vi "1. Empty String to Typical data types.vi"() -> ()   [LabVIEW 2017]
doc: "### Overview\nDemonstrates how the CSM API supports converting empty strings to typical data types. In most cases, an empty string is converted to the numerical value connected to the reference data type. The following is an exception:\n\n- **String data type:** An empty string converts to an empty string.\n\n### Introduction\nDemonstrates converting various empty strings to typical data types. Pay special attention to the exception regarding the String data type. The front panel displays the reference values and the converted values for comparison.\n### Steps\n\n- step1: For all common types, an empty string converts to the numerical value connected to the reference data type.\n- step2: For the String data type, an empty string converts to an empty string.\n- step3: For the Timestamp data type, an empty string converts to the current time."
uses:
  2bb2f873-33e8-4fbc-8df2-f8c3b892e92f.vi
  d59d594f-6358-4fe9-a0ea-ade5f599e91a.vi
  177f037c-d6c1-4684-97ba-f775e359171c.vi
  f8914412-5770-4d7c-8ed9-34d3b6c64140.vi
  83982d16-e29d-493a-892c-93b6b063dd3a.vi
  40fc1cc9-77e3-4a14-9bb9-de70462c7f35.vi
  81b41104-5ca5-45e9-a143-87b761583821.vi
  38ed8c4c-bfe5-4ceb-af5c-8de10cee5e52.vi
  a345cc07-d10f-4275-8a18-17707c3f89e9.vi
  cabc4c38-4671-4b03-9489-31c074b0dc0c.vi
  efc68658-e21b-4998-9bfe-a9de0054dd82.vi
  0842be61-58c2-4c06-9355-20aaf40be817.vi
  a49a9376-e1ff-4fda-bff8-7fdb6b491f6f.vi
  addons/API-String-Arugments-Support/_Support/Convert API String Arguments to Data(variant).vi
panel:
  out "timestamp":T1={"Argument String"="", "Type"=timestamp(0 s since 1904-01-01), "Retrieved TimeStamp"=timestamp(3839278850.481537 s since 1904-01-01)}
  out "2d double array":T2={"Empty API String"="", "2D DBL"=[[3.12, 4.113, 2.3, 5.0, 5.0, 2.3, 4.11, 5.0]], "Retrieved Data"=[[3.12, 4.113, 2.3, 5.0, 5.0, 2.3, 4.11, 5.0]]}
  out "cluster array":T3={"Empty API String"="", "Cluster Array"=[{"Name"="", "Child"={"Name"="ddd"}, "Bool"=FALSE}, {"Name"="ddd", "Child"={"Name"=""}, "Bool"=TRUE}], "Retrieved Data"=[{"Name"="", "Child"={"Name"="ddd"}, "Bool"=FALSE}, {"Name"="ddd", "Child"={"Name"=""}, "Bool"=TRUE}]}
  out "cluster":T4={"Empty API String"="", "Cluster"={"Name"="abc", "Child"={"Name"="ddd"}, "Bool"=FALSE}, "Retrieved Data"={"Name"="abc", "Child"={"Name"="ddd"}, "Bool"=FALSE}}
  out "1d dbl":T5={"Empty API String"="", "1D DBL"=[3.12, 4.11, 5.0], "Retrieved Data"=[3.12, 4.11, 5.0]}
  out "enum3":T6={"Empty API String"="", "Enum"=enum."2 - bbbb", "Retrieved Data"=enum."1 - aaaa"}
  out "enum2":T6
  out "enum1":T7={"Empty API String"="", "Enum"=enum."ccccc", "Retrieved Data"=enum."aaaa"}
  out "dbl":T8={"Empty API String"="", "DBL"=3.1415926, "Retrieved Data"=3.1415926}
  out "i32":T9={"Empty API String"="", "I32"=66, "Retrieved Data"=66}
  out "boolean":T10={"Empty API String"="", "Boolean"=TRUE, "Retrieved Data"=TRUE}
  out "string":T11={"Empty API String"="", "String"="abcd", "Retrieved Data"=""}
  out "path":T12={"Empty API String"="", "Path"=path "C:/ni-rt/data/a/2023.07.25", "Retrieved Data"=path "C:/ni-rt/data/a/2023.07.25"}
  # "#CSM-Example Overview\nDemonstrates how the CSM API supports converting empty strings to typical data types. In most cases, an empty string is converted to the numerical value connected to the reference data type. The following is an exception:\n\n- **String data type:** An empty string converts to an empty string."
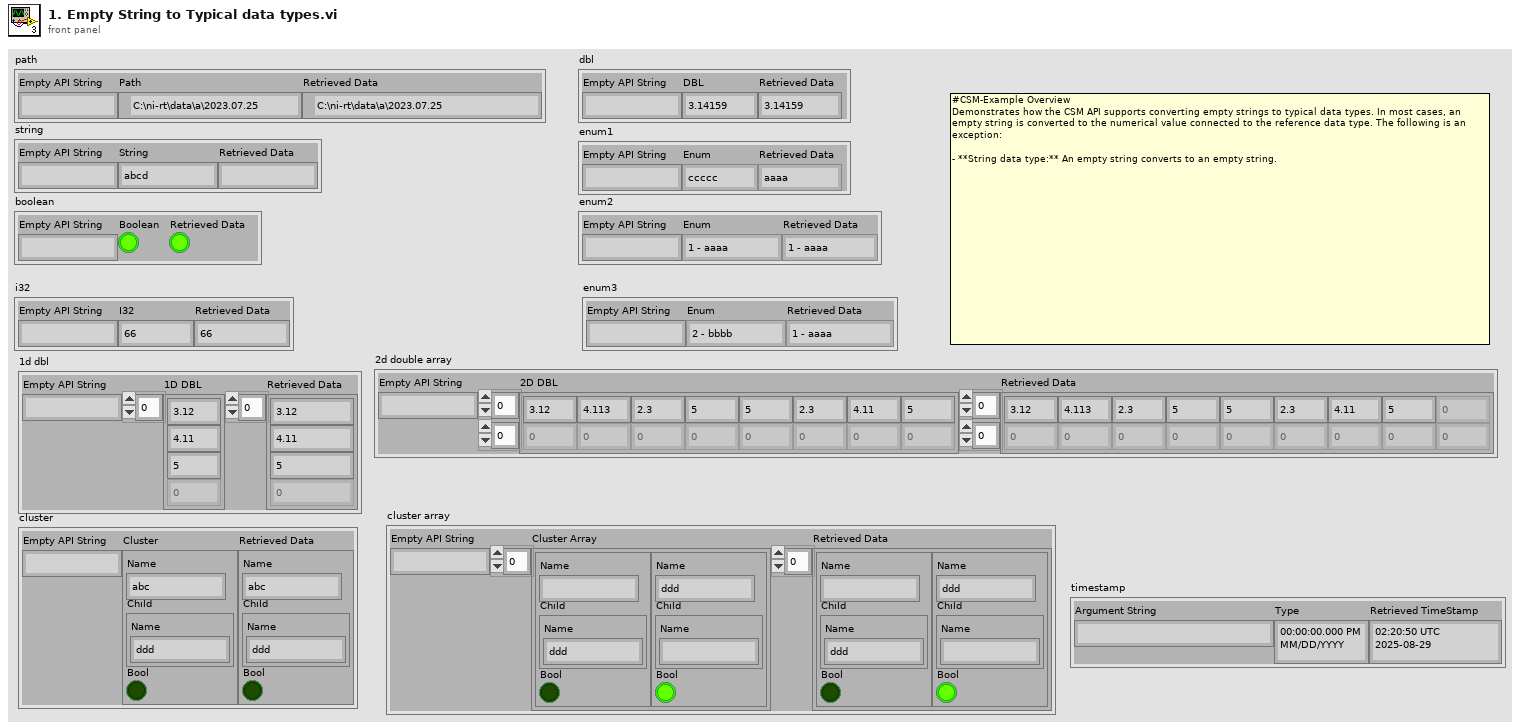
[diagram p1: front panel]
types:
  T1 = cluster{"Argument String":string, "Type":timestamp, "Retrieved TimeStamp":timestamp}
  T2 = cluster{"Empty API String":string, "2D DBL":dbl[][], "Retrieved Data":dbl[][]}
  T3 = cluster{"Empty API String":string, "Cluster Array":cluster{"Name":string, "Child":cluster{"Name":string}, "Bool":bool}[], "Retrieved Data":cluster{"Name":string, "Child":cluster{"Name":string}, "Bool":bool}[]}
  T4 = cluster{"Empty API String":string, "Cluster":cluster{"Name":string, "Child":cluster{"Name":string}, "Bool":bool}, "Retrieved Data":cluster{"Name":string, "Child":cluster{"Name":string}, "Bool":bool}}
  T5 = cluster{"Empty API String":string, "1D DBL":dbl[], "Retrieved Data":dbl[]}
  T6 = cluster{"Empty API String":string, "Enum":enum16{"1 - aaaa", "2 - bbbb", "555 - ccccc"}, "Retrieved Data":enum16{"1 - aaaa", "2 - bbbb", "555 - ccccc"}}
  T7 = cluster{"Empty API String":string, "Enum":enum16{"aaaa", "bbbb", "ccccc"}, "Retrieved Data":enum16{"aaaa", "bbbb", "ccccc"}}
  T8 = cluster{"Empty API String":string, "DBL":dbl, "Retrieved Data":dbl}
  T9 = cluster{"Empty API String":string, "I32":i32, "Retrieved Data":i32}
  T10 = cluster{"Empty API String":string, "Boolean":bool, "Retrieved Data":bool}
  T11 = cluster{"Empty API String":string, "String":string, "Retrieved Data":string}
  T12 = cluster{"Empty API String":string, "Path":path, "Retrieved Data":path}
  T13 = cluster{"Name":string, "Child":cluster{"Name":string}, "Bool":bool}[]
  T14 = cluster{"Name":string, "Child":cluster{"Name":string}, "Bool":bool}
  T15 = cluster{"Empty API String":string, "Data 9":path, "Data":path}
  T16 = cluster{"Empty API String":string, "Data 1":string, "Data":string}
  T17 = cluster{"Empty API String":string, "Data 2":bool, "Data":bool}
  T18 = cluster{"Empty API String":string, "Data 3":i32, "Data":i32}
  T19 = cluster{"Empty API String":string, "Data 4":dbl, "Data":dbl}
  T20 = cluster{"Empty API String":string, "Data 5":enum16{"aaaa", "bbbb", "ccccc"}, "Data":enum16{"aaaa", "bbbb", "ccccc"}}
  T21 = cluster{"Empty API String":string, "Data 6":enum16{"1 - aaaa", "2 - bbbb", "555 - ccccc"}, "Data":enum16{"1 - aaaa", "2 - bbbb", "555 - ccccc"}}
  T22 = cluster{"Empty API String":string, "Data 7":enum16{"1 - aaaa", "2 - bbbb", "555 - ccccc"}, "Data":enum16{"1 - aaaa", "2 - bbbb", "555 - ccccc"}}
  T23 = cluster{"Empty API String":string, "Data 4":dbl[], "Data":dbl[]}
  T24 = cluster{"Empty API String":string, "Data 8":cluster{"Name":string, "Child":cluster{"Name":string}, "Bool":bool}, "Data":cluster{"Name":string, "Child":cluster{"Name":string}, "Bool":bool}}
  T25 = cluster{"Empty API String":string, "Data 10":cluster{"Name":string, "Child":cluster{"Name":string}, "Bool":bool}[], "Data":cluster{"Name":string, "Child":cluster{"Name":string}, "Bool":bool}[]}
  T26 = cluster{"Empty API String":string, "Data 11":dbl[][], "Data":dbl[][]}
  T27 = cluster{"Empty String":string, "Type":timestamp, "Data":timestamp}
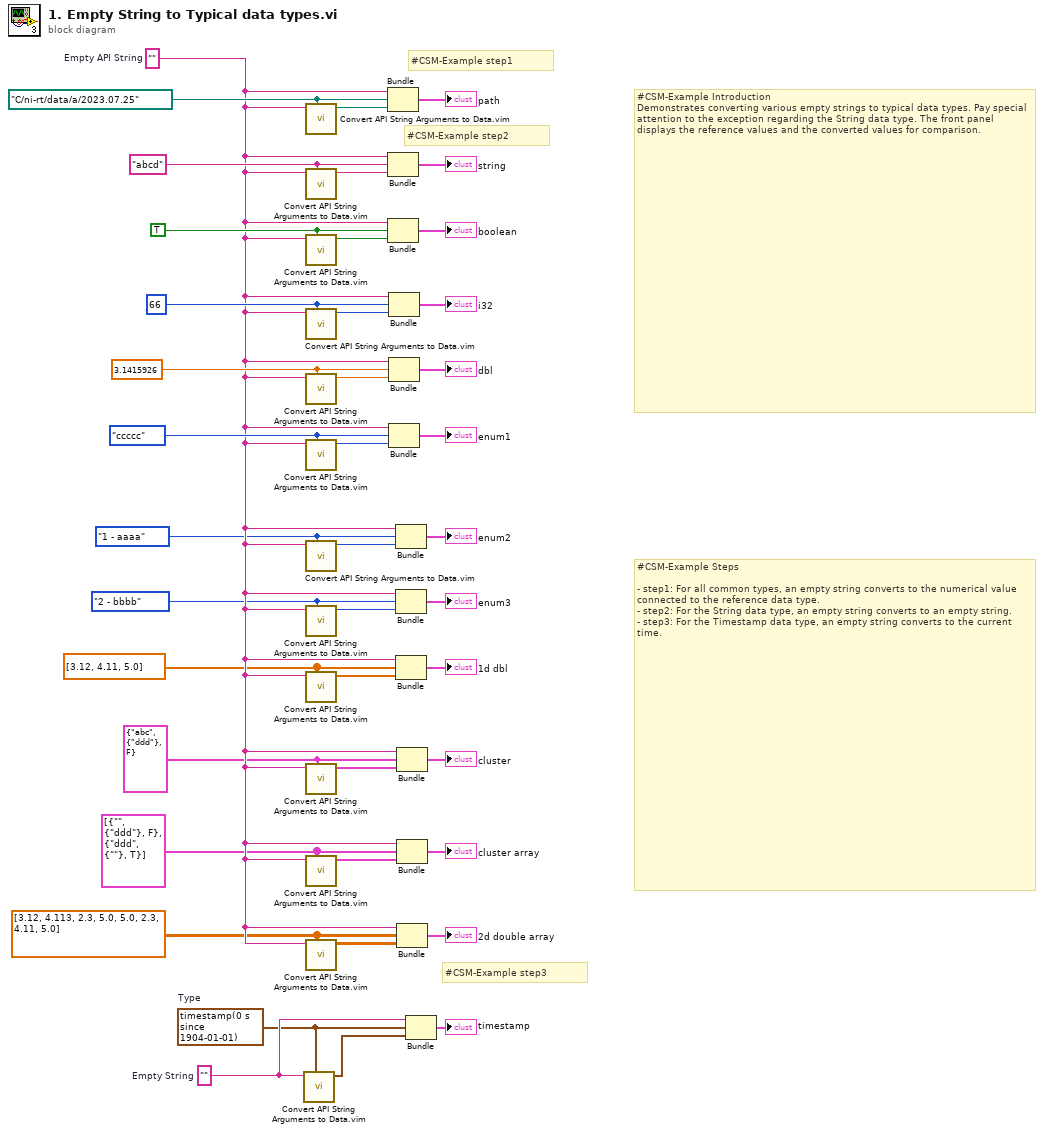
[diagram p0: block diagram]
diagram:
  w4 = ""  # Empty String
  w3 = timestamp(0 s since 1904-01-01)  # Type
  w11 = dbl[][] [[3.12, 4.113, 2.3, 5.0, 5.0, 2.3, 4.11, 5.0]] ("Data 11")
  w12 = T13 [{"Name"="", "Child"={"Name"="ddd"}, "Bool"=FALSE}, {"Name"="ddd", "Child"={"Name"=""}, "Bool"=TRUE}] ("Data 10")
  w13 = T14 {"Name"="abc", "Child"={"Name"="ddd"}, "Bool"=FALSE} ("Data 8")
  w14 = dbl[] [3.12, 4.11, 5.0] ("Data 4")
  w15 = enum16{"1 - aaaa", "2 - bbbb", "555 - ccccc"}."2 - bbbb" ("Data 7")
  w16 = enum16{"1 - aaaa", "2 - bbbb", "555 - ccccc"}."1 - aaaa" ("Data 6")
  w27 = enum16{"aaaa", "bbbb", "ccccc"}."ccccc" ("Data 5")
  w28 = 3.1415926 ("Data 4")
  w29 = 66 ("Data 3")
  w34 = TRUE ("Data 2")
  w38 = "abcd" ("Data 1")
  w41 = path "C:/ni-rt/data/a/2023.07.25" ("Data 9")
  w17 = ""  # Empty API String
  # "#CSM-Example step3"
  # "#CSM-Example step1"
  # "#CSM-Example Steps\n\n- step1: For all common types, an empty string converts to the numerical value connected to the reference data type.\n- step2: For the String data type, an empty string converts to an empty string.\n- step3: For the Timestamp data type, an empty string converts to the current time."
  # "#CSM-Example step2"
  # "#CSM-Example Introduction\nDemonstrates converting various empty strings to typical data types. Pay special attention to the exception regarding the String data type. The front panel displays the reference values and the converted values for comparison."
  n1 = call "Convert API String Arguments to Data.vim"("Reference Type"=w3, "API String"=w4) -> ("Data"=w2:timestamp)  [unwired: 6 in, 1 out]
  n2 = call "Convert API String Arguments to Data.vim"("Reference Type"=w41, "API String"=w17) -> ("Data"=w40:path)  [unwired: 6 in, 1 out]
  n3 = call "Convert API String Arguments to Data.vim"("Reference Type"=w38, "API String"=w17) -> ("Data"=w37:string)  [unwired: 6 in, 1 out]
  n4 = call "Convert API String Arguments to Data.vim"("Reference Type"=w34, "API String"=w17) -> ("Data"=w35:bool)  [unwired: 6 in, 1 out]
  n5 = call "Convert API String Arguments to Data.vim"("Reference Type"=w29, "API String"=w17) -> ("Data"=w30:i32)  [unwired: 6 in, 1 out]
  n6 = call "Convert API String Arguments to Data.vim"("Reference Type"=w28, "API String"=w17) -> ("Data"=w31:dbl)  [unwired: 6 in, 1 out]
  n7 = call "Convert API String Arguments to Data.vim"("Reference Type"=w27, "API String"=w17) -> ("Data"=w32:enum16{"aaaa", "bbbb", "ccccc"})  [unwired: 6 in, 1 out]
  n8 = call "Convert API String Arguments to Data.vim"("Reference Type"=w16, "API String"=w17) -> ("Data"=w18:enum16{"1 - aaaa", "2 - bbbb", "555 - ccccc"})  [unwired: 6 in, 1 out]
  n9 = call "Convert API String Arguments to Data.vim"("Reference Type"=w15, "API String"=w17) -> ("Data"=w19:enum16{"1 - aaaa", "2 - bbbb", "555 - ccccc"})  [unwired: 6 in, 1 out]
  n10 = call "Convert API String Arguments to Data.vim"("Reference Type"=w14, "API String"=w17) -> ("Data"=w20:dbl[])  [unwired: 6 in, 1 out]
  n11 = call "Convert API String Arguments to Data.vim"("Reference Type"=w13, "API String"=w17) -> ("Data"=w23:T14)  [unwired: 6 in, 1 out]
  n12 = call "Convert API String Arguments to Data.vim"("Reference Type"=w12, "API String"=w17) -> ("Data"=w22:T13)  [unwired: 6 in, 1 out]
  n13 = call "Convert API String Arguments to Data.vim"("Reference Type"=w11, "API String"=w17) -> ("Data"=w21:dbl[][])  [unwired: 6 in, 1 out]
  n14 = Bundle("Empty API String"=w17, "Data 9"=w41, "Data"=w40) -> (→"path":T15)  [unwired: 1 in]
  n15 = Bundle("Empty API String"=w17, "Data 1"=w38, "Data"=w37) -> (→"string":T16)  [unwired: 1 in]
  n16 = Bundle("Empty API String"=w17, "Data 2"=w34, "Data"=w35) -> (→"boolean":T17)  [unwired: 1 in]
  n17 = Bundle("Empty API String"=w17, "Data 3"=w29, "Data"=w30) -> (→"i32":T18)  [unwired: 1 in]
  n18 = Bundle("Empty API String"=w17, "Data 4"=w28, "Data"=w31) -> (→"dbl":T19)  [unwired: 1 in]
  n19 = Bundle("Empty API String"=w17, "Data 5"=w27, "Data"=w32) -> (→"enum1":T20)  [unwired: 1 in]
  n20 = Bundle("Empty API String"=w17, "Data 6"=w16, "Data"=w18) -> (→"enum2":T21)  [unwired: 1 in]
  n21 = Bundle("Empty API String"=w17, "Data 7"=w15, "Data"=w19) -> (→"enum3":T22)  [unwired: 1 in]
  n22 = Bundle("Empty API String"=w17, "Data 4"=w14, "Data"=w20) -> (→"1d dbl":T23)  [unwired: 1 in]
  n23 = Bundle("Empty API String"=w17, "Data 8"=w13, "Data"=w23) -> (→"cluster":T24)  [unwired: 1 in]
  n24 = Bundle("Empty API String"=w17, "Data 10"=w12, "Data"=w22) -> (→"cluster array":T25)  [unwired: 1 in]
  n25 = Bundle("Empty API String"=w17, "Data 11"=w11, "Data"=w21) -> (→"2d double array":T26)  [unwired: 1 in]
  n26 = Bundle("Empty String"=w4, "Type"=w3, "Data"=w2) -> (→"timestamp":T27)  [unwired: 1 in]
